vi "our rocket league.vi"(11 "Axes":dbl[](array[numeric])) -> (1 "upper limit":dbl, 2 "upper limit 2":dbl, 3 "upper limit 3":dbl)   [LabVIEW 2019]
uses:
  <vilib>/Rock Robotics/Network Tables/NT Read String.vi
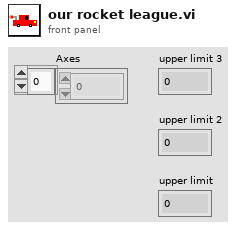
[diagram p1: front panel]
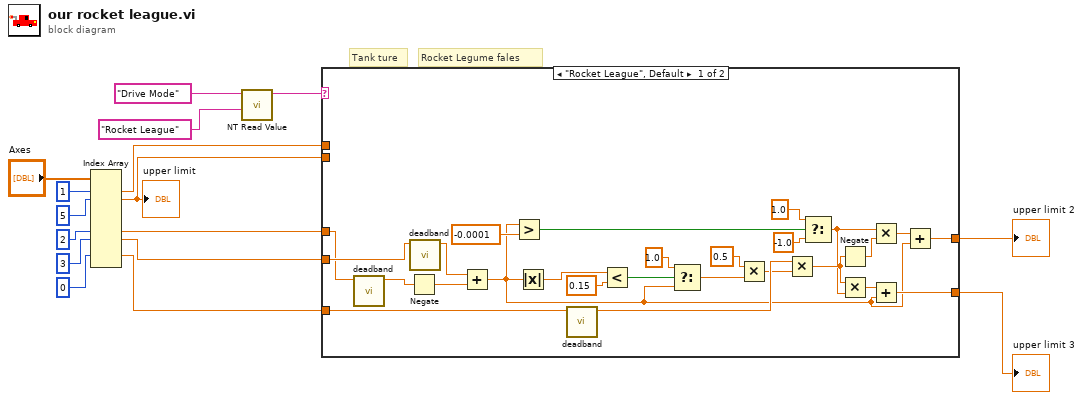
[diagram p0: block diagram]
diagram:
  # "Rocket Legume fales"
  # "Tank ture"
  n1 = Index Array(array="Axes", index #1=1 ("index"), index #2=5 ("index"), index #6=2 ("index"), index #7=3 ("index"), index #9=0 ("index")) -> (element #1=w4:dbl, element #2=w16:dbl, element #6=w9:dbl, element #7=w10:dbl, element #9=w15:dbl)  [unwired: 5 in, 5 out]
  "upper limit" <- w16
  n2 = call-poly <vilib>:"NT Read Value.vi"("Default Value"="Rocket League", "Name"="Drive Mode") -> ("String"=w12:string)  [unwired: 8 in, 1 out]
  n3 = case shown="\"Rocket League\", Default" w12 {
    tunnel: w4 -> [_ w44]
    tunnel: w16 -> [_ w43]
    tunnel: [w26 w44] -> w5
    tunnel: [w27 w43] -> w6
    tunnel: w9 -> [w24 _]
    tunnel: w10 -> [w25 _]
    tunnel: w15 -> [w23 _]
    frame "Rocket League", Default {
      n4 = call "deadband.vi"("Joystick Value"=w24) -> ("Val"=w41:dbl)  [unwired: 10 in]
      n5 = Negate(x=w41) -> (-x=w39:dbl)
      n6 = call "deadband.vi"("Joystick Value"=w25) -> ("Val"=w40:dbl)  [unwired: 10 in]
      n7 = Add(x=w40, y=w39) -> (x+y=w21:dbl)
      n8 = Greater?(x=w21, y=-0.0001) -> (0:w37:bool)
      n9 = Absolute Value(x=w21) -> (abs(x)=w20:dbl)
      n10 = call "deadband.vi"("Joystick Value"=w23) -> ("Val"=w42:dbl)  [unwired: 10 in]
      n11 = Less?(x=w20, y=0.15) -> (x < y?=w18:bool)
      n12 = Select(t=1.0, s=w18, f=w21) -> (s? t:f=w17:dbl)
      n13 = Multiply(x=0.5, y=w17) -> (x*y=w29:dbl)
      n14 = Multiply(x=w42, y=w29) -> (x*y=w34:dbl)
      n15 = Select(t=1.0, s=w37, f=-1.0) -> (s? t:f=w32:dbl)
      n16 = Negate(x=w34) -> (-x=w31:dbl)
      n17 = Multiply(x=w34, y=w32) -> (x*y=w33:dbl)
      n18 = Multiply(x=w32, y=w31) -> (x*y=w30:dbl)
      n19 = Add(x=w33, y=w21) -> (x+y=w26:dbl)
      n20 = Add(x=w30, y=w21) -> (x+y=w27:dbl)
    }
    frame "Tank" {
    }
  }
  "upper limit 2" <- w6
  "upper limit 3" <- w5
